vi "Yaw adjust (SubVI).vi"(11 "X":sgl) -> (1 "Boolean":bool, 2 "Numeric":dbl, 3 "Boolean 2":bool)   [LabVIEW 2014]
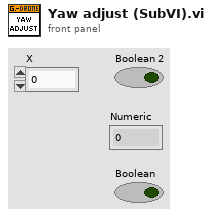
[diagram p1: front panel]
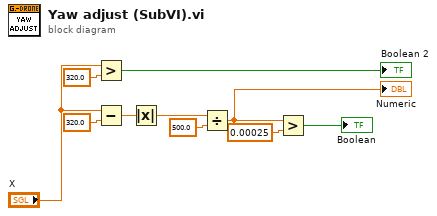
[diagram p0: block diagram]
diagram:
  n1 = Greater?(x="X", y=320.0) -> (0:→"Boolean 2":bool)
  n2 = Subtract(x="X", y=320.0) -> (x-y=w3:dbl)
  n3 = Absolute Value(x=w3) -> (abs(x)=w4:dbl)
  n4 = Divide(x=w4, y=500.0) -> (x/y=w8:dbl)
  "Numeric" <- w8
  n5 = Greater?(x=w8, y=0.00025) -> (0:→"Boolean":bool)
